vi "Actor Core.vi"(8 "error in":errorcluster, 11 "Nested in":refnum<class "Chef UI.lvclass">) -> (0 "error out":errorcluster, 3 "Actor out":refnum<class "Actor.lvclass">)   [LabVIEW 2024, in "Chef UI.lvlib" / "Chef UI.lvclass"]
doc: "(<B>Filename</B>: Actor Framework.lvlib:Actor.lvclass:Actor Core.vi)\n\nReceives messages to the actor, reacts to them, and initiates any error handling that may shut the actor down.\n\nDescendant classes may override this VI to append parallel tasks for the actor to complete while it handles messages. Overrides use the Call Parent Method node."
uses:
  Chef UI.lvclass
  C:/Program Files/National Instruments/LabVIEW 2024/vi.lib/ActorFramework/Actor/Actor.lvclass
  <vilib>/ActorFramework/Actor/Actor.lvclass
  Chef State/Init/Init.lvclass
  <vilib>/ActorFramework/Actor/Actor.lvclass/Actor.ctl
  <vilib>/ActorFramework/Message Enqueuer/Message Enqueuer.lvclass/Message Enqueuer.ctl
  Chef UI.lvclass/Chef UI.ctl
  <vilib>/ActorFramework/Message Enqueuer/Init from Existing Queue.vi
  <vilib>/ActorFramework/Message Enqueuer/Enqueue.vi
  <vilib>/ActorFramework/Stop Msg/Stop Msg.lvclass
  C:/Program Files/National Instruments/LabVIEW 2024/vi.lib/ActorFramework/Message/Message.lvclass
  <vilib>/ActorFramework/Message Priority Queue/Priority Enqueue.vi
  <vilib>/ActorFramework/Message Enqueuer/Message Enqueuer.lvclass
  C:/Users/burakkorkmaz/Desktop/PROJE/actor-state-machine/Chef UI/Chef UI.lvclass
  C:/Users/burakkorkmaz/Desktop/PROJE/actor-state-machine/Chef UI Logic/Chef UI Logic/Chef UI Logic.lvclass
  C:/Users/burakkorkmaz/Desktop/PROJE/actor-state-machine/Chef State/Chef State/Chef State.lvclass
  C:/Program Files/National Instruments/LabVIEW 2024/vi.lib/NI/Actors/State Actor/State Actor/State Actor.lvclass
  C:/Users/burakkorkmaz/Desktop/PROJE/actor-state-machine/Chef State/Init/Init.lvclass
panel:
  out "Log":string
  in  "Stop Button":bool
  in  "Start Button":bool
  out "Count":dbl
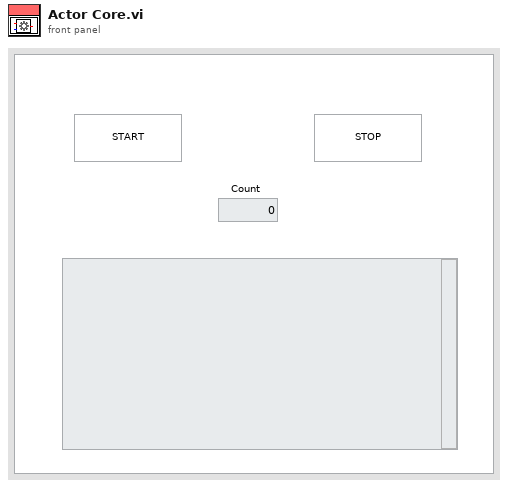
[diagram p1: front panel]
types:
  T1 = cluster{"Stop":refnum<user-event>, "Log":refnum<user-event>, "Count":refnum<user-event>}
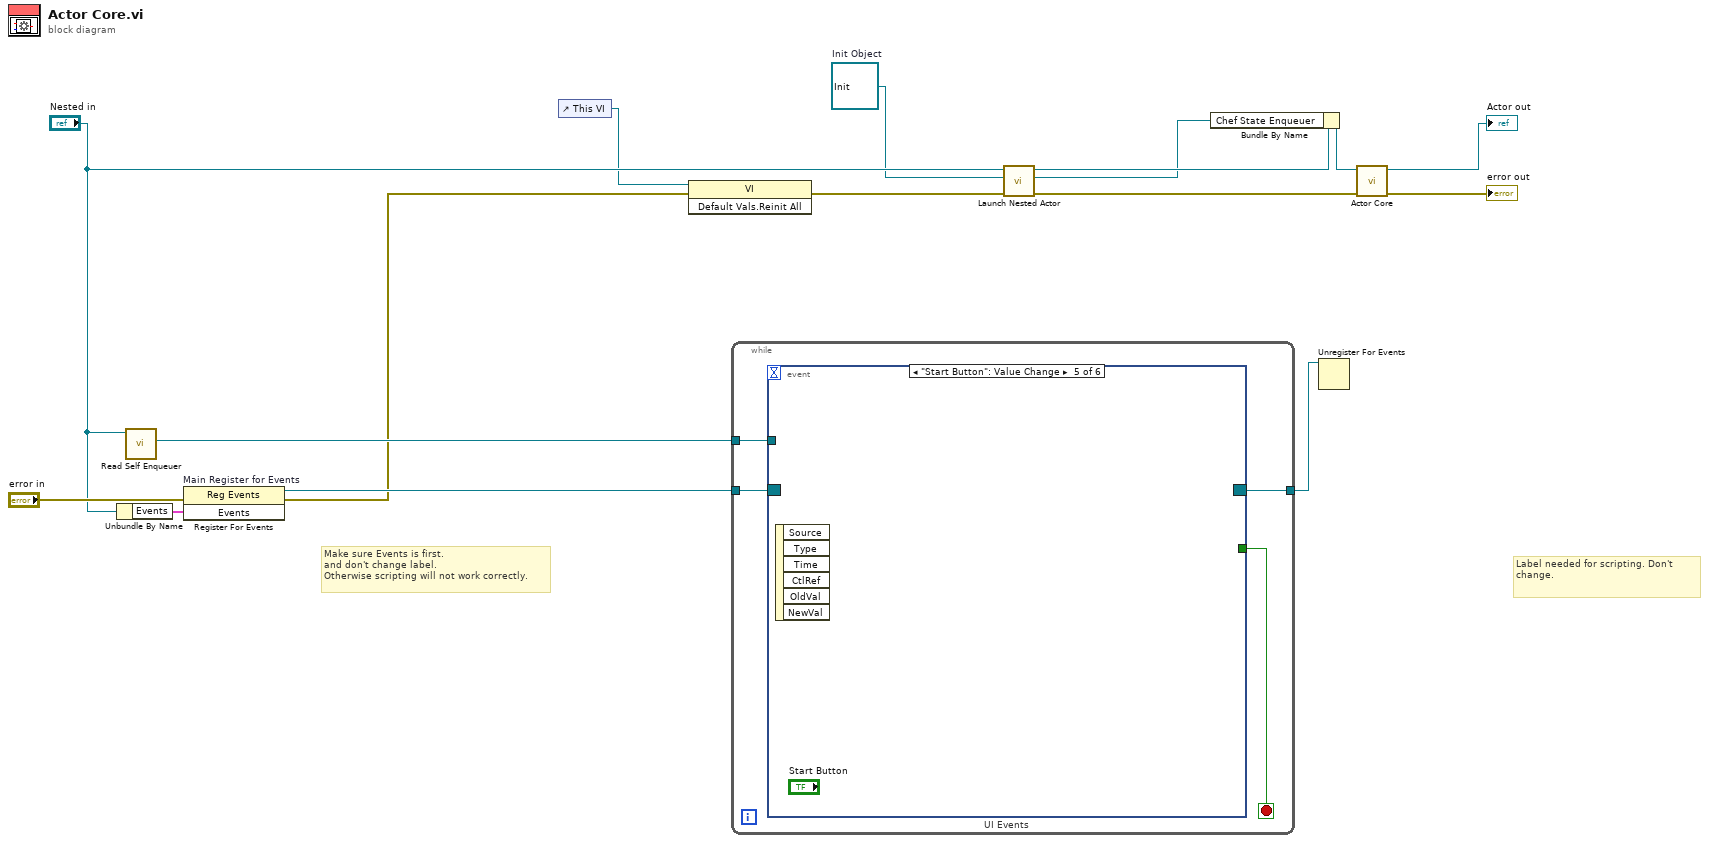
[diagram p0: block diagram]
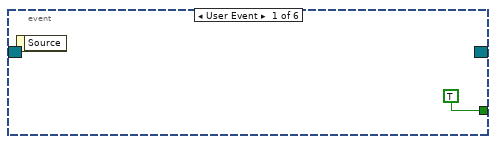
[diagram p2: hidden frame]
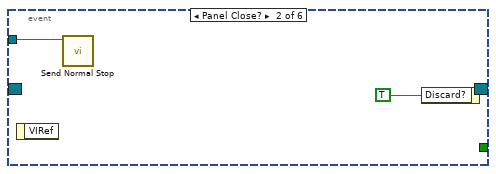
[diagram p3: hidden frame]
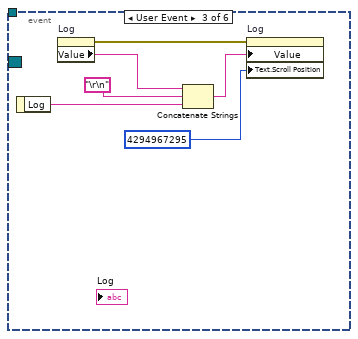
[diagram p4: hidden frame]
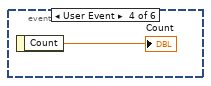
[diagram p5: hidden frame]
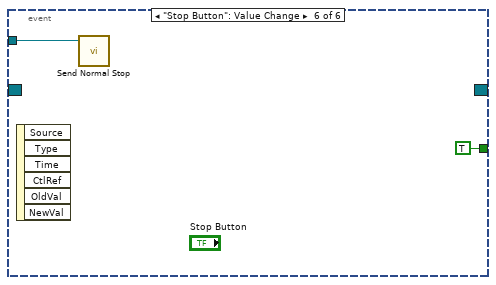
[diagram p6: hidden frame]
diagram:
  w6 = refnum<class "Init.lvclass"> refnum  # Init Object
  # "Label needed for scripting. Don't change."
  # "Make sure Events is first.\nand don't change label.\nOtherwise scripting will not work correctly."
  n1 = Unbundle By Name("Nested in") -> ("Events"=w13:T1)
  n2 = call <vilib>:"Read Self Enqueuer.vi"("Actor"="Nested in") -> ("Self Enqueuer"=w11:refnum<class "Message Enqueuer.lvclass">)  [unwired: 10 in]
  n3 = register-events "Main Register for Events"(error in="error in", w13) -> (reference out=w14:refnum<event-registration>, error out=w2:errorcluster)  [unwired: 1 in]
  n4 = control-ref of="This VI"() -> (w3:refnum<vi>)
  n5 = invoke class="VI" method="Default Vals.Reinit All"(reference=w3, error in=w2) -> (error out=w1:errorcluster)  [unwired: 1 in, 2 out]
  n6 = while {
    tunnel: w14 -> [w20]
    tunnel: [w18] -> w12
    tunnel: w11 -> [w17]
    stop <- w19 stop-if-true
    n7 = event "UI Events" shown="[4] \"Start Button\": Value Change" {
      selector: w20 -> [_ _ _ _ _ _]
      dyn-events: [_ _ _ _ _ _] -> w18
      timeout: _ -> [_ _ _ _ _ _]
      tunnel: [TRUE _ _ _ _ TRUE] -> w19
      tunnel: w17 -> [_ w22 _ _ _ w32]
      event User Event {
        n8 = event-data() -> ()  [unwired: 1 in, 1 out]
      }
      event Panel Close? {
        n9 = event-data() -> ()  [unwired: 1 in, 1 out]
        n10 = call <vilib>:"Send Normal Stop.vi"("Message Enqueuer"=w22) -> ()  [unwired: 10 in, 1 out]
        n11 = event-data("Discard?"=TRUE) -> ()  [unwired: 1 in, 1 out]
      }
      event User Event {
        n12 = event-data() -> ("Log"=w28:string)  [unwired: 1 in]
        n13 = property on="Log" class="Str"() -> (error out=w24:errorcluster, "Value"=w29:string)  [unwired: 2 in, 1 out]
        n14 = Concatenate Strings(w29, "\r\n", w28) -> (w26:string)
        n15 = property on="Log" class="Str"(error in=w24, "Value"=w26, "Text.Scroll Position"=i64 4294967295) -> ()  [unwired: 1 in, 2 out]
      }
      event User Event {
        n16 = event-data() -> ("Count"=→"Count":dbl)  [unwired: 1 in]
      }
      event "Start Button": Value Change {
        n17 = event-data() -> ()  [unwired: 1 in, 6 out]
      }
      event "Stop Button": Value Change {
        n18 = event-data() -> ()  [unwired: 1 in, 6 out]
        n19 = call <vilib>:"Send Normal Stop.vi"("Message Enqueuer"=w32) -> ()  [unwired: 10 in, 1 out]
      }
    }
  }
  n20 = call <vilib>:"Launch Nested Actor.vi"("error in (no error)"=w1, "Nested Actor"=w6, "Caller Actor in"="Nested in") -> ("error out"=w7:errorcluster, "Nested Actor's Enqueuer"=w4:refnum<class "Message Enqueuer.lvclass">, "Caller Actor out"=w8:refnum<class "Chef UI.lvclass">)  [unwired: 6 in]
  n21 = Bundle By Name(cluster=w8, "Chef State Enqueuer"=w4) -> (w5:refnum<class "Chef UI.lvclass">)
  n22 = Unregister For Events(event registration refnum=w12) -> ()  [unwired: 1 in, 1 out]
  n23 = call-parent "Actor Core.vi"("error in"=w7, "Actor in"=w5) -> ("error out"=→"error out":errorcluster, "Actor out"=→"Actor out":refnum<class "Actor.lvclass">)  [unwired: 8 in]
